vi "Configure Voltage Coupling.vi"(8 "error in (no error)":errorcluster, 9 "Enable Coupling (T: Enable)":bool=TRUE, 10 "Channel (1:1)":u16(ring)=1 items=["1"=1, "2"=2], 11 "VISA resource name":refnum<visa-resource-name>) -> (0 "error out":errorcluster, 3 "VISA resource name out":refnum<visa-resource-name>)   [LabVIEW 2015, in "Agilent 3352X Series.lvlib"]
doc: "Enables voltage coupling to set the instrument's amplitude, offset, range, load, and units on both channels to the same value, and keep them the same. \nWhen this Voltage Coupling is turned ON, the specified channel will send its present setting to the other channel."
uses:
  <instrlib>/Agilent 3352X Series/Agilent 3352X Series.lvlib
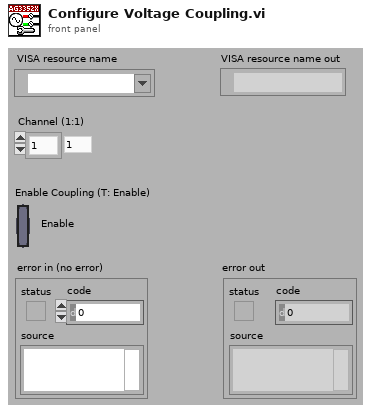
[diagram p1: front panel]
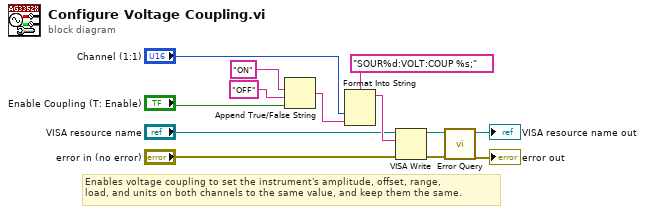
[diagram p0: block diagram]
diagram:
  # "Enables voltage coupling to set the instrument's amplitude, offset, range, \nload, and units on both channels to the same value, and keep them the same."
  n1 = Append True/False String(1:"Enable Coupling (T: Enable)", 2:"OFF", 3:"ON") -> (0:w8:string)  [unwired: 1 out]
  n2 = Format Into String(format string="SOUR%d:VOLT:COUP %s;", "Channel (1:1)", w8) -> (resulting string=w7:string)  [unwired: 2 in, 1 out]
  n3 = VISA Write(VISA resource name="VISA resource name", write buffer=w7, error in (no error)="error in (no error)") -> (VISA resource name out=w4:refnum<visa-resource-name>, error out=w3:errorcluster)  [unwired: 1 out]
  n4 = call <instrlib>:"Error Query.vi"("error in (no error)"=w3, "VISA resource name"=w4) -> ("error out"=→"error out":errorcluster, "VISA resource name out"=→"VISA resource name out":refnum<visa-resource-name>)  [unwired: 8 out]
